vi "SetROI.vi"(7 "error in (no error)":errorcluster, 9 "SizeIn":T1, 10 "reference in":refnum<k24>) -> (0 "error out":errorcluster, 2 "SizeOut":T1, 3 "reference out":refnum<k24>)   [LabVIEW 2018]
uses:
  C:/Program Files/National Instruments/LabVIEW 2018/instr.lib/IDS/ueye.NET/uEyeDotNet.dll
  instr.lib/IDS/ueye.NET/uEyeDotNet.dll
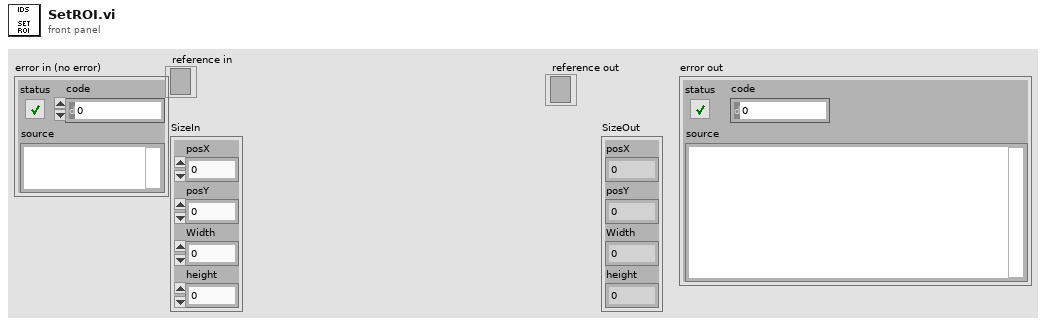
[diagram p1: front panel]
types:
  T1 = cluster{"posX":i32, "posY":i32, "Width":i32, "height":i32}
  T2 = cluster{"upper limit":dbl, "lower limit":dbl, "increment":dbl}
  T3 = cluster{"s32PosX":i32, "s32PosY":i32, "s32Width":i32, "s32Height":i32}
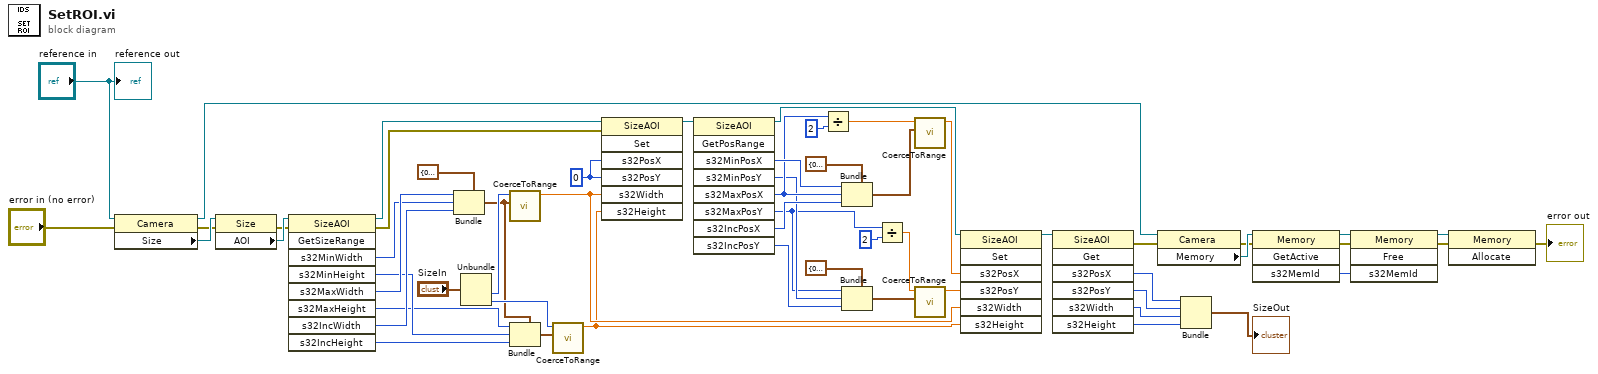
[diagram p0: block diagram]
diagram:
  w26 = 0 ("s32PosY")
  n1 = property class="Camera"(reference="reference in", error in="error in (no error)") -> (reference out=w46:refnum<k24>, error out=w37:errorcluster, "Size"=w56:refnum<k24>)
  n2 = property class="Size"(reference=w56, error in=w37) -> (error out=w36:errorcluster, "AOI"=w55:refnum<k24>)  [unwired: 1 out]
  n3 = invoke class="SizeAOI" method="GetSizeRange"(reference=w55, error in=w36) -> (reference out=w25:refnum<k24>, error out=w24:errorcluster, "s32MinWidth"=w34:i32, "s32MinHeight"=w31:i32, "s32MaxWidth"=w35:i32, "s32MaxHeight"=w30:i32, "s32IncWidth"=w33:i32, "s32IncHeight"=w29:i32)  [unwired: 7 in, 1 out]
  n4 = Bundle(cluster=T2 {"upper limit"=0.0, "lower limit"=0.0, "increment"=0.0} ("Range"), "upper limit"=w35, "lower limit"=w34, "increment"=w33) -> (w21:T2)
  n5 = Unbundle("SizeIn") -> ("Width"=w32:i32, "height"=w27:i32)  [unwired: 2 out]
  n6 = call <userlib>:"CoerceToRange.vi"("Range"=w21, "input"=w32) -> ("coerced"=w4:dbl)  [unwired: 9 in]
  n7 = Bundle(cluster=w21, "upper limit"=w30, "lower limit"=w31, "increment"=w29) -> (w28:T2)
  n8 = call <userlib>:"CoerceToRange.vi"("Range"=w28, "input"=w27) -> ("coerced"=w3:dbl)  [unwired: 9 in]
  n9 = invoke class="SizeAOI" method="Set"(reference=w25, error in=w24, "s32PosX"=w26, "s32PosY"=w26, "s32Width"=w4, "s32Height"=w3) -> (reference out=w23:refnum<k24>)  [unwired: 1 in, 6 out]
  n10 = invoke class="SizeAOI" method="GetPosRange"(reference=w23) -> (reference out=w2:refnum<k24>, "s32MinPosX"=w19:i32, "s32MinPosY"=w12:i32, "s32MaxPosX"=w16:i32, "s32MaxPosY"=w9:i32, "s32IncPosX"=w18:i32, "s32IncPosY"=w11:i32)  [unwired: 8 in, 2 out]
  n11 = Divide(x=w16, y=2) -> (x/y=w14:dbl)
  n12 = Bundle(cluster=T2 {"upper limit"=0.0, "lower limit"=0.0, "increment"=0.0} ("Range"), "upper limit"=w19, "lower limit"=w16, "increment"=w18) -> (w17:T2)
  n13 = Bundle(cluster=T2 {"upper limit"=0.0, "lower limit"=0.0, "increment"=0.0} ("Range"), "upper limit"=w9, "lower limit"=w12, "increment"=w11) -> (w7:T2)
  n14 = Divide(x=w9, y=2) -> (x/y=w8:dbl)
  n15 = call <userlib>:"CoerceToRange.vi"("Range"=w17, "input"=w14) -> ("coerced"=w6:dbl)  [unwired: 9 in]
  n16 = call <userlib>:"CoerceToRange.vi"("Range"=w7, "input"=w8) -> ("coerced"=w5:dbl)  [unwired: 9 in]
  n17 = invoke class="SizeAOI" method="Set"(reference=w2, "s32PosX"=w6, "s32PosY"=w5, "s32Width"=w4, "s32Height"=w3) -> (reference out=w1:refnum<k24>)  [unwired: 2 in, 6 out]
  n18 = invoke class="SizeAOI" method="Get"(reference=w1) -> (error out=w47:errorcluster, "s32PosX"=w54:i32, "s32PosY"=w53:i32, "s32Width"=w52:i32, "s32Height"=w51:i32)  [unwired: 6 in, 2 out]
  n19 = property class="Camera"(reference=w46, error in=w47) -> (error out=w43:errorcluster, "Memory"=w45:refnum<k24>)  [unwired: 1 out]
  n20 = Bundle("s32PosX"=w54, "s32PosY"=w53, "s32Width"=w52, "s32Height"=w51) -> (→"SizeOut":T3)  [unwired: 1 in]
  n21 = invoke class="Memory" method="GetActive"(reference=w45, error in=w43) -> (reference out=w40:refnum<k24>, error out=w42:errorcluster, "s32MemId"=w44:i32)  [unwired: 2 in, 1 out]
  n22 = invoke class="Memory" method="Free"(reference=w40, error in=w42, "s32MemId"=w44) -> (reference out=w41:refnum<k24>, error out=w39:errorcluster)  [unwired: 1 in, 2 out]
  n23 = invoke class="Memory" method="Allocate"(reference=w41, error in=w39) -> (error out=→"error out":errorcluster)  [unwired: 1 in, 2 out]
  "reference out" <- "reference in"
